vi "EnumerateElements.vi"(8 "error in (no error)":errorcluster, 10 "Qualified Name":string, 11 "ConfigManager.Cache in":refnum<class "ConfigManager.Cache.lvclass">) -> (0 "error out":errorcluster, 2 "keys":string[](array[string]), 3 "ConfigManager.Cache out":refnum<class "ConfigManager.Cache.lvclass">)   [LabVIEW 2013, in "SMOConfig.lvlib" / "ConfigManager.Cache.lvclass"]
uses:
  ConfigManager.Cache.lvclass
  ConfigManager.Cache.lvclass/ConfigManager.Cache.ctl
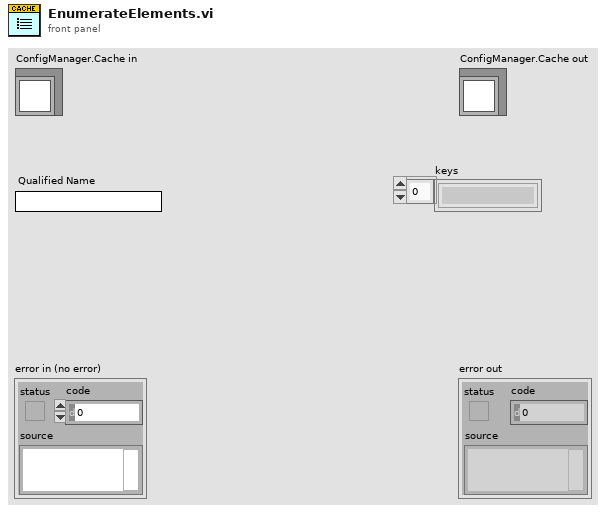
[diagram p1: front panel]
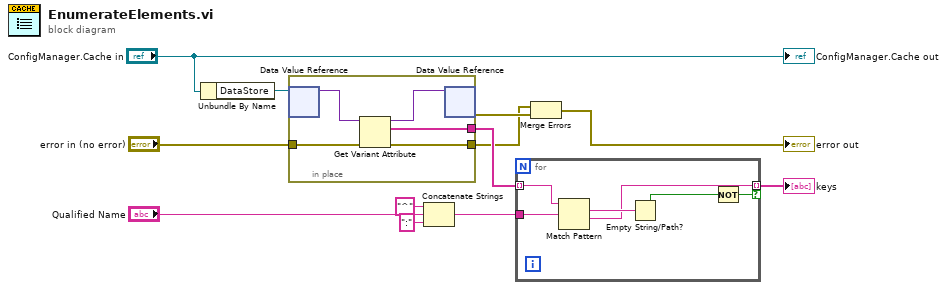
[diagram p0: block diagram]
diagram:
  n1 = Unbundle By Name("ConfigManager.Cache in") -> ("DataStore"=w1:refnum<data-value>)
  n2 = in-place {
    in-place-border: "error in (no error)" -> [w17]
    in-place-border: [w16] -> w3
    in-place-border: [w15] -> w11
    n3 = in-place-dvr #1(w1) -> (w14:variant)  [unwired: 1 out]
    n4 = Get Variant Attribute(Variant=w14, error in=w17) -> (duplicate Variant=w13:variant, names=w15:string[], error out=w16:errorcluster)  [unwired: 2 in, 1 out]
    n5 = in-place-dvr #1(w13) -> (w5:errorcluster)  [unwired: 1 out]
  }
  n6 = Concatenate Strings("^" ("string"), "Qualified Name", ":" ("string")) -> (w9:string)
  n7 = for {
    tunnel: w11 -> [w18] mode=indexing
    tunnel: w9 -> [w23]
    tunnel: [w19] -> w8 mode=indexing if=w20
    n8 = Match Pattern(string=w18, regular expression=w23) -> (match substring=w22:string, after substring=w19:string)  [unwired: 1 in, 2 out]
    n9 = Empty String/Path?(string/path=w22) -> (empty?=w21:bool)
    n10 = Not(x=w21) -> (.not. x?=w20:bool)
  }
  "keys" <- w8
  n11 = Merge Errors(w3, w5) -> (→"error out":errorcluster)
  "ConfigManager.Cache out" <- "ConfigManager.Cache in"
